vi "Initialize_Lithography.vi"(8 "error in":errorcluster, 11 "Application":refnum<k7>) -> (0 "error out":errorcluster, 3 "lithography_Offsets":cluster{"X":dbl, "Y":dbl})   [LabVIEW 2016]
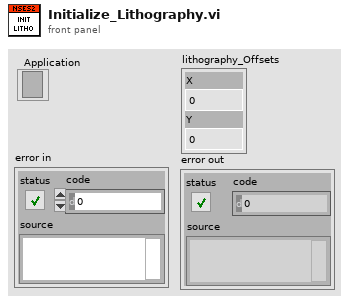
[diagram p1: front panel]
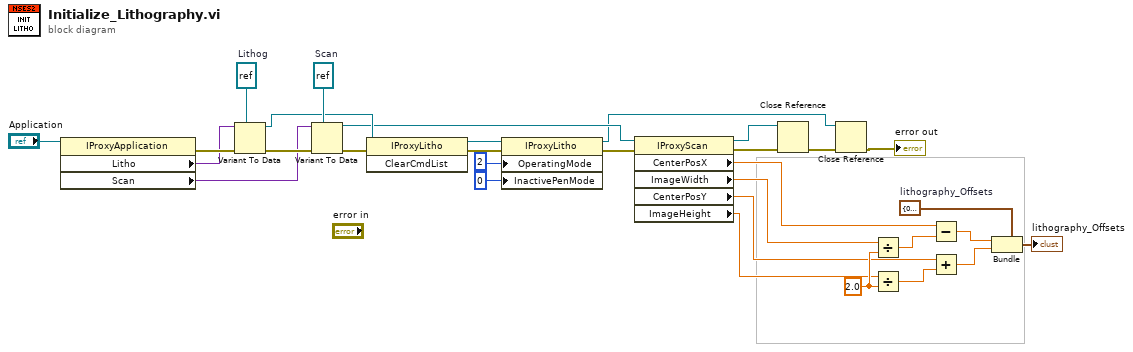
[diagram p0: block diagram]
diagram:
  w5 = cluster{"X":dbl, "Y":dbl} {"X"=0.0, "Y"=0.0}  # lithography_Offsets
  w11 = 2.0 ("y")
  w28 = refnum<k7> refnum  # Lithog
  w27 = refnum<k7> refnum  # Scan
  n1 = property class="IProxyApplication"(reference="Application") -> (error out=w30:errorcluster, "Litho"=w26:variant, "Scan"=w25:variant)  [unwired: 1 in, 1 out]
  n2 = Variant To Data(error in=w30, type=w28, Variant=w26) -> (data=w23:refnum<k7>, error out=w29:errorcluster)
  n3 = Variant To Data(error in=w29, type=w27, Variant=w25) -> (data=w17:refnum<k7>, error out=w24:errorcluster)
  n4 = invoke class="IProxyLitho" method="ClearCmdList"(reference=w23, error in=w24) -> (reference out=w21:refnum<k7>, error out=w22:errorcluster)  [unwired: 1 in, 1 out]
  n5 = property class="IProxyLitho"(reference=w21, error in=w22, "OperatingMode"=2, "InactivePenMode"=0) -> (reference out=w13:refnum<k7>, error out=w18:errorcluster)
  n6 = property class="IProxyScan"(reference=w17, error in=w18) -> (reference out=w16:refnum<k7>, error out=w15:errorcluster, "CenterPosX"=w6:dbl, "ImageWidth"=w7:dbl, "CenterPosY"=w8:dbl, "ImageHeight"=w9:dbl)
  n7 = Close Reference(reference=w16, error in (no error)=w15) -> (error out=w14:errorcluster)
  n8 = Close Reference(reference=w13, error in (no error)=w14) -> (error out=→"error out":errorcluster)
  n9 = Divide(x=w7, y=w11) -> (x/y=w10:dbl)
  n10 = Divide(x=w9, y=w11) -> (x/y=w12:dbl)
  n11 = Subtract(x=w6, y=w10) -> (x-y=w4:dbl)
  n12 = Add(x=w8, y=w12) -> (x+y=w3:dbl)
  n13 = Bundle(cluster=w5, "X"=w4, "Y"=w3) -> (→"lithography_Offsets":cluster{"X":dbl, "Y":dbl})
